vi "Reboot.vi"(7 "LabVIEW Web Service Request":refnum<class "Web Request.lvclass">) -> ()   [LabVIEW 2014]
uses:
  <vilib>/wsapi/Web Request.lvclass
  <vilib>/nisyscfg/Close (System).vi
  <vilib>/nisyscfg/nisyscfg.lvlib
panel:
  # "Use the Web Service Request input terminal to call the VIs on the Web Services palette. Do not remove it from the connector pane unless you don't need access to the palette."
  # "Each additional control wired to the connector pane will be available as an input in the URL. To include an indicator in terminal-mode output (the default setting), it must also be wired to the connector pane."
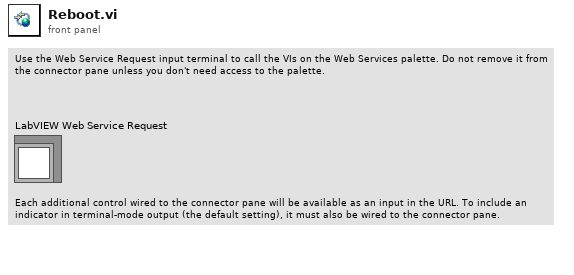
[diagram p1: front panel]
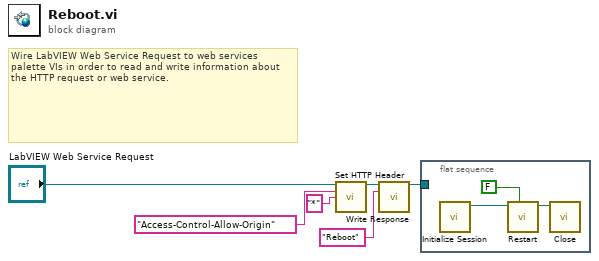
[diagram p0: block diagram]
diagram:
  # "Wire LabVIEW Web Service Request to web services palette VIs in order to read and write information about the HTTP request or web service."
  n1 = call <vilib>:"Set HTTP Header.vi"("LabVIEW Web Service Request"="LabVIEW Web Service Request", "header"="Access-Control-Allow-Origin", "header value"="*") -> ("LabVIEW Web Service Request out"=w1:refnum<class "Web Request.lvclass">)  [unwired: 11 in, 1 out]
  n2 = call <vilib>:"Write Response.vi"("LabVIEW Web Service Request"=w1, "response string"="Reboot") -> ("LabVIEW Web Service Request out"=w5:refnum<class "Web Request.lvclass">)  [unwired: 12 in, 1 out]
  n3 = flat-sequence {
    tunnel: w5 -> [_]
    frame #0 {
      n4 = call <vilib>:"Initialize Session.vi"() -> ("Session out"=w9:refnum<k21>)  [unwired: 10 in, 1 out]
      n5 = call <vilib>:"Restart.vi"("Wait Until Complete (T)"=FALSE, "Session in"=w9) -> ("Session out"=w8:refnum<k21>)  [unwired: 7 in, 2 out]
      n6 = call-poly <vilib>:"Close.vi"("Session in"=w8) -> ()  [unwired: 10 in, 1 out]
    }
  }
